vi "Test.vi"(7 "Label (VI Title)":string, 8 "error in (no error)":errorcluster, 11 "Type":variant) -> (0 "error out":errorcluster)   [LabVIEW 2018, in "JSON to LVConstant Test.lvlib"]
uses:
  JSON to LVConstant Test.lvlib
  9a1572e7-135a-41bf-ab18-c450e40867d5.vi
  <vilib>/JDP Science/JSONtext/Variant to JSON Text.vi
  <vilib>/addons/_JKI Toolkits/Caraya/classes/Assert/Assert Equal Type_Variant.vi
  <vilib>/JDP Science/JSONtext/LVClass Serializer/JSONtext LVClass Serializer.lvclass
  Source/SLL Scripting/SLL Scripting.lvlib
  <vilib>/addons/_JKI Toolkits/Caraya/classes/Assert/Assert.lvclass
  <vilib>/addons/_JKI Toolkits/Caraya/classes/Test/Test.lvclass
  <vilib>/JDP Science/JSONtext/JSONtext.lvlib
  <vilib>/addons/_JKI Toolkits/Caraya/classes/Assert/Assert Equal Value_Variant.vi
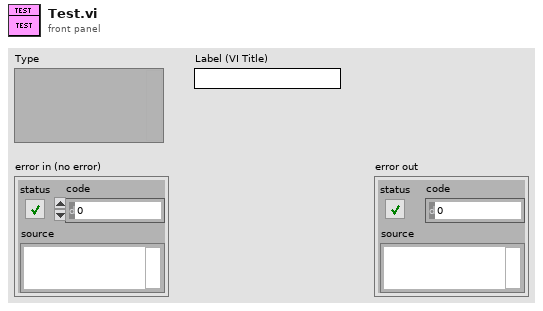
[diagram p1: front panel]
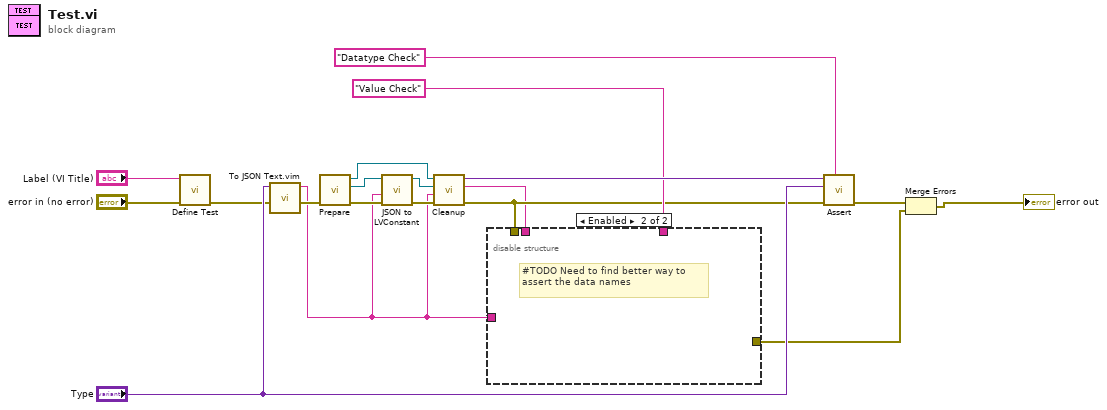
[diagram p0: block diagram]
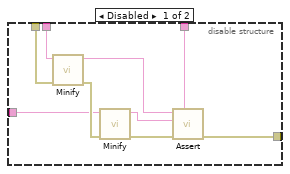
[diagram p2: hidden frame]
diagram:
  n1 = call <vilib>:"Define Test.vi"("error in (no error)"="error in (no error)", "Label (VI Title)"="Label (VI Title)") -> ("error out"=w7:errorcluster)  [unwired: 9 in]
  n2 = call "To JSON Text.vim"("error in (no error)"=w7, "Anything"="Type") -> ("error out"=w13:errorcluster, "<JSON>"=w2:string)  [unwired: 8 in]
  n3 = call "Prepare.vi"("error in (no error)"=w13) -> ("error out"=w12:errorcluster, "Owner"=w15:refnum<vi>, "vi refnum"=w16:refnum<vi>)  [unwired: 8 in]
  n4 = call "JSON to LVConstant.vi"("error in (no error)"=w12, "<JSON>"=w2, "owner refnum in"=w15) -> ("error out"=w11:errorcluster, "owner refnum out"=w17:refnum<vi>)  [unwired: 7 in]
  n5 = call "Cleanup.vi"("error in (no error)"=w11, "JSON"=w2, "Owner"=w17, "vi refnum"=w16) -> ("error out"=w3:errorcluster, "JSON out"=w1:string, "Type out"=w19:variant)  [unwired: 5 in]
  n6 = disable-structure "Diagram Disable Structure" shown="Enabled" {
    disable-tunnel: "Value Check" ("Label (VI Title)") -> [w28 _]
    disable-tunnel: [w27 _] -> w4
    disable-tunnel: w3 -> [w26 _]
    disable-tunnel: w2 -> [w21 _]
    disable-tunnel: w1 -> [w20 _]
    frame Disabled {
      n7 = call <vilib>:"Minify.vi"("error in (no error)"=w26, "JSON"=w20) -> ("error out"=w23:errorcluster, "<JSON>"=w25:string)  [unwired: 7 in, 1 out]
      n8 = call <vilib>:"Minify.vi"("error in (no error)"=w23, "JSON"=w21) -> ("error out"=w22:errorcluster, "<JSON>"=w24:string)  [unwired: 7 in, 1 out]
      n9 = call-poly <vilib>:"Assert.vi"("Label"=w28, "error in (no error)"=w22, "Y"=w24, "X"=w25) -> ("error out"=w27:errorcluster)  [unwired: 7 in]
    }
    frame Enabled {
      # "#TODO Need to find better way to assert the data names"
    }
  }
  n10 = call-poly <vilib>:"Assert.vi"("Label"="Datatype Check" ("Label (VI Title)"), "error in (no error)"=w3, "Y"="Type", "X"=w19) -> ("error out"=w18:errorcluster)  [unwired: 7 in]
  n11 = Merge Errors(w18, w4) -> (→"error out":errorcluster)
